vi "Teleop.vi"(10 "Match Info":T1={"Autonomous Elapsed Seconds"=0.0, "TeleOp Elapsed Seconds"=0.0, "Disabled Elapsed Seconds"=0.0, "Visited Autonomous"=FALSE, "Visited TeleOp"=FALSE, "Visited Disabled"=FALSE, "Autonomous Settings"={"Autonomous Style"=enum."Independent", "VI Refnum"=refnum}}, 11 "Call Context":T2) -> ()   [LabVIEW 2019]
doc: "This VI is called for each TeleOp packet received from the DS where the robot is not disabled. It is often used to read from the joysticks and update I/O or to update setpoints for timed control loops. It should complete and return within 20 milliseconds or it may miss DS packets."
uses:
  <vilib>/Rock Robotics/WPI/DriverStation/WPI_DriverStationDerivedRobotMode.ctl
  <vilib>/Rock Robotics/WPI/DriverStation/WPI_DriverStationMatch Info.ctl
  <vilib>/Rock Robotics/WPI/ThirdParty/Phoenix-LabVIEW/Motor Controller/Controls/CTRE_Phoenix_MotorControl_ControlMode.ctl
  <vilib>/Rock Robotics/WPI/Solenoid/WPI_SolenoidValue.ctl
  <vilib>/Rock Robotics/WPI/Utilities/WPI_GetSetVariantRefNum.vi
  <vilib>/Rock Robotics/Network Tables/NT Read Number.vi
  <vilib>/addons/control/pid/pid.llb/PID (DBL).vi
  <vilib>/Rock Robotics/Network Tables/NT Write Number.vi
  <vilib>/Rock Robotics/WPI/ThirdParty/Phoenix-LabVIEW/Motor Controller/Get/CTRE_Phoenix_MotorController_GetSelectedSensorData.vi
  <vilib>/Rock Robotics/Network Tables/NT Write Boolean.vi
  <vilib>/functionblocks/Bistables/SR Bistable/SR Bistable.vi
  <vilib>/Rock Robotics/Network Tables/NT Write Numeric Array.vi
  <vilib>/Rock Robotics/WPI/Solenoid/WPI_SolenoidSetEnum.vi
  <vilib>/functionblocks/FB Core/FB Core.xnode
  <vilib>/Rock Robotics/Network Tables/NT Read Boolean.vi
  <vilib>/addons/control/pid/NI_PID_pid.lvlib
  <vilib>/functionblocks/NI_FunctionBlock Libraries.lvlib
  <vilib>/Rock Robotics/Network Tables/NT Write Boolean Array.vi
panel:
  out "Sample Slider 0":dbl(slide) scale=0.0..5.0
  out "Sample Boolean 1":bool
  out "Sample Boolean 0":bool
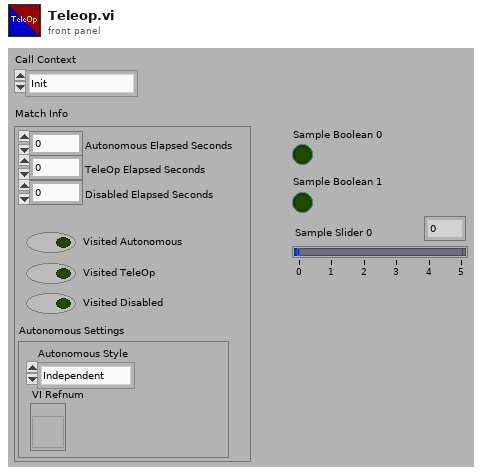
[diagram p1: front panel]
types:
  T1 = typedef "WPI_DriverStationMatch Info.ctl" = cluster{"Autonomous Elapsed Seconds":dbl, "TeleOp Elapsed Seconds":dbl, "Disabled Elapsed Seconds":dbl, "Visited Autonomous":bool, "Visited TeleOp":bool, "Visited Disabled":bool, "Autonomous Settings":cluster{"Autonomous Style":enum16{"Iterative", "Independent"}, "VI Refnum":refnum<vi>}}
  T2 = typedef "WPI_DriverStationDerivedRobotMode.ctl" = enum16{"Init", "Execute", "Stop"}
  T3 = typedef "CTRE_Phoenix_MotorControl_ControlMode.ctl" = u16
  T4 = typedef "WPI_JoystickDevRef.ctl" = cluster{"Device":T5}
  T5 = typedef "WPI_JoystickDeviceEnum.ctl" = enum16{"USB 0", "USB 1", "USB 2", "USB 3", "USB 4", "USB 5"}
  T6 = typedef "WPI_RobotDriveDevRef.ctl" = cluster{"DevStatus":errorcluster, "Motors[]":T7[], "Square Inputs":bool, "Max Output":dbl}
  T7 = typedef "WPI_MotorControlDeviceRef.ctl" = cluster{"DeviceStatus":errorcluster, "Type":T8, "PWM":cluster{"PWM Channel":T9, "DeadBand":T10}, "CAN":cluster{"Device Number":u8, "SetOutput VI Ref":variant, "GetOutput VI Ref":variant, "Enable VI Ref":variant, "Disable VI Ref":variant, "Data":variant}, "Invert":bool, "DIO PWM":cluster{"PWM \"Enable\" Channel":T9, "DIOChannel":T11, "PWM Rate":dbl}}
  T8 = typedef "WPI_MotorControlType.ctl" = enum16{"PWM", "CAN", "DIO PWM"}
  T9 = typedef "FPGA_DIOPWMChannel.ctl" = enum8{"PWM 0", "PWM 1", "PWM 2", "PWM 3", "PWM 4", "PWM 5", "PWM 6", "PWM 7", "PWM 8", "PWM 9", "PWM MXP 0", "PWM MXP 1", "PWM MXP 2", "PWM MXP 3", "PWM MXP 4", "PWM MXP 5", "PWM MXP 6", "PWM MXP 7", "PWM MXP 8", "PWM MXP 9", "Invalid"}
  T10 = typedef "WPI_PWMDeadband.ctl" = cluster{"Name":string, "maxPositivePwm":i32, "minPositivePwm":i32, "centerPwm":i32, "maxNegativePwm":i32, "minNegativePwm":i32, "angularRange":u16}
  T11 = typedef "FPGA_DIOChannel.ctl" = enum8{"DIO 0", "DIO 1", "DIO 2", "DIO 3", "DIO 4", "DIO 5", "DIO 6", "DIO 7", "DIO 8", "DIO 9", "DIO MXP 0", "DIO MXP 1", "DIO MXP 2", "DIO MXP 3", "DIO MXP 4", "DIO MXP 5", "DIO MXP 6", "DIO MXP 7", "DIO MXP 8", "DIO MXP 9", "DIO MXP 10", "DIO MXP 11", "DIO MXP 12", "DIO MXP 13", "DIO MXP 14", "DIO MXP 15", "SPI Port CS1", "SPI Port CS2", "SPI Port CS3", "SPI Port MISO", "SPI Port MOSI", "Invalid"}
  T12 = cluster{"Buttons[0]":bool, "Buttons[1]":bool, "Buttons[2]":bool, "Buttons[3]":bool, "Buttons[4]":bool, "Buttons[5]":bool, "Buttons[6]":bool, "Buttons[7]":bool, "Buttons[8]":bool, "Buttons[9]":bool}
  T13 = cluster{"Axes[0]":dbl, "Axes[1]":dbl, "Axes[2]":dbl, "Axes[3]":dbl, "Axes[4]":dbl, "Axes[5]":dbl, "Axes[6]":dbl, "Axes[7]":dbl, "Axes[8]":dbl}
  T14 = cluster{"proportional gain (Kc)":dbl, "integral time (Ti, min)":dbl, "derivative time (Td, min)":dbl}
  T15 = typedef "WPI_ServoDeviceRef.ctl" = cluster{"DeviceStatus":errorcluster, "PWM Channel":T9, "DeadBand":T10}
  T16 = typedef "WPI_SolenoidDevRef.ctl" = cluster{"DevStatus":errorcluster, "Pneumatics Control Module":u8, "Forward Solenoid Channel":T17, "Reverse Solenoid Channel":T17}
  T17 = typedef "WPI_SolenoidChannel.ctl" = enum8{"Solenoid 0", "Solenoid 1", "Solenoid 2", "Solenoid 3", "Solenoid 4", "Solenoid 5", "Solenoid 6", "Solenoid 7", "Invalid"}
  T18 = typedef "WPI_SolenoidValue.ctl" = enum16{"Off", "On", "Forward", "Reverse"}
  T19 = typedef "WPI_SwitchDevRef.ctl" = cluster{"DevStatus":errorcluster, "DIO Channel":T11, "CntIndex":T20, "Normally Closed":bool}
  T20 = typedef "FPGA_CounterCtrSystemIndex.ctl" = enum8{"Ctr 0", "Ctr 1", "Ctr 2", "Ctr 3", "Ctr 4", "Ctr 5", "Ctr 6", "Ctr 7", "Invalid"}
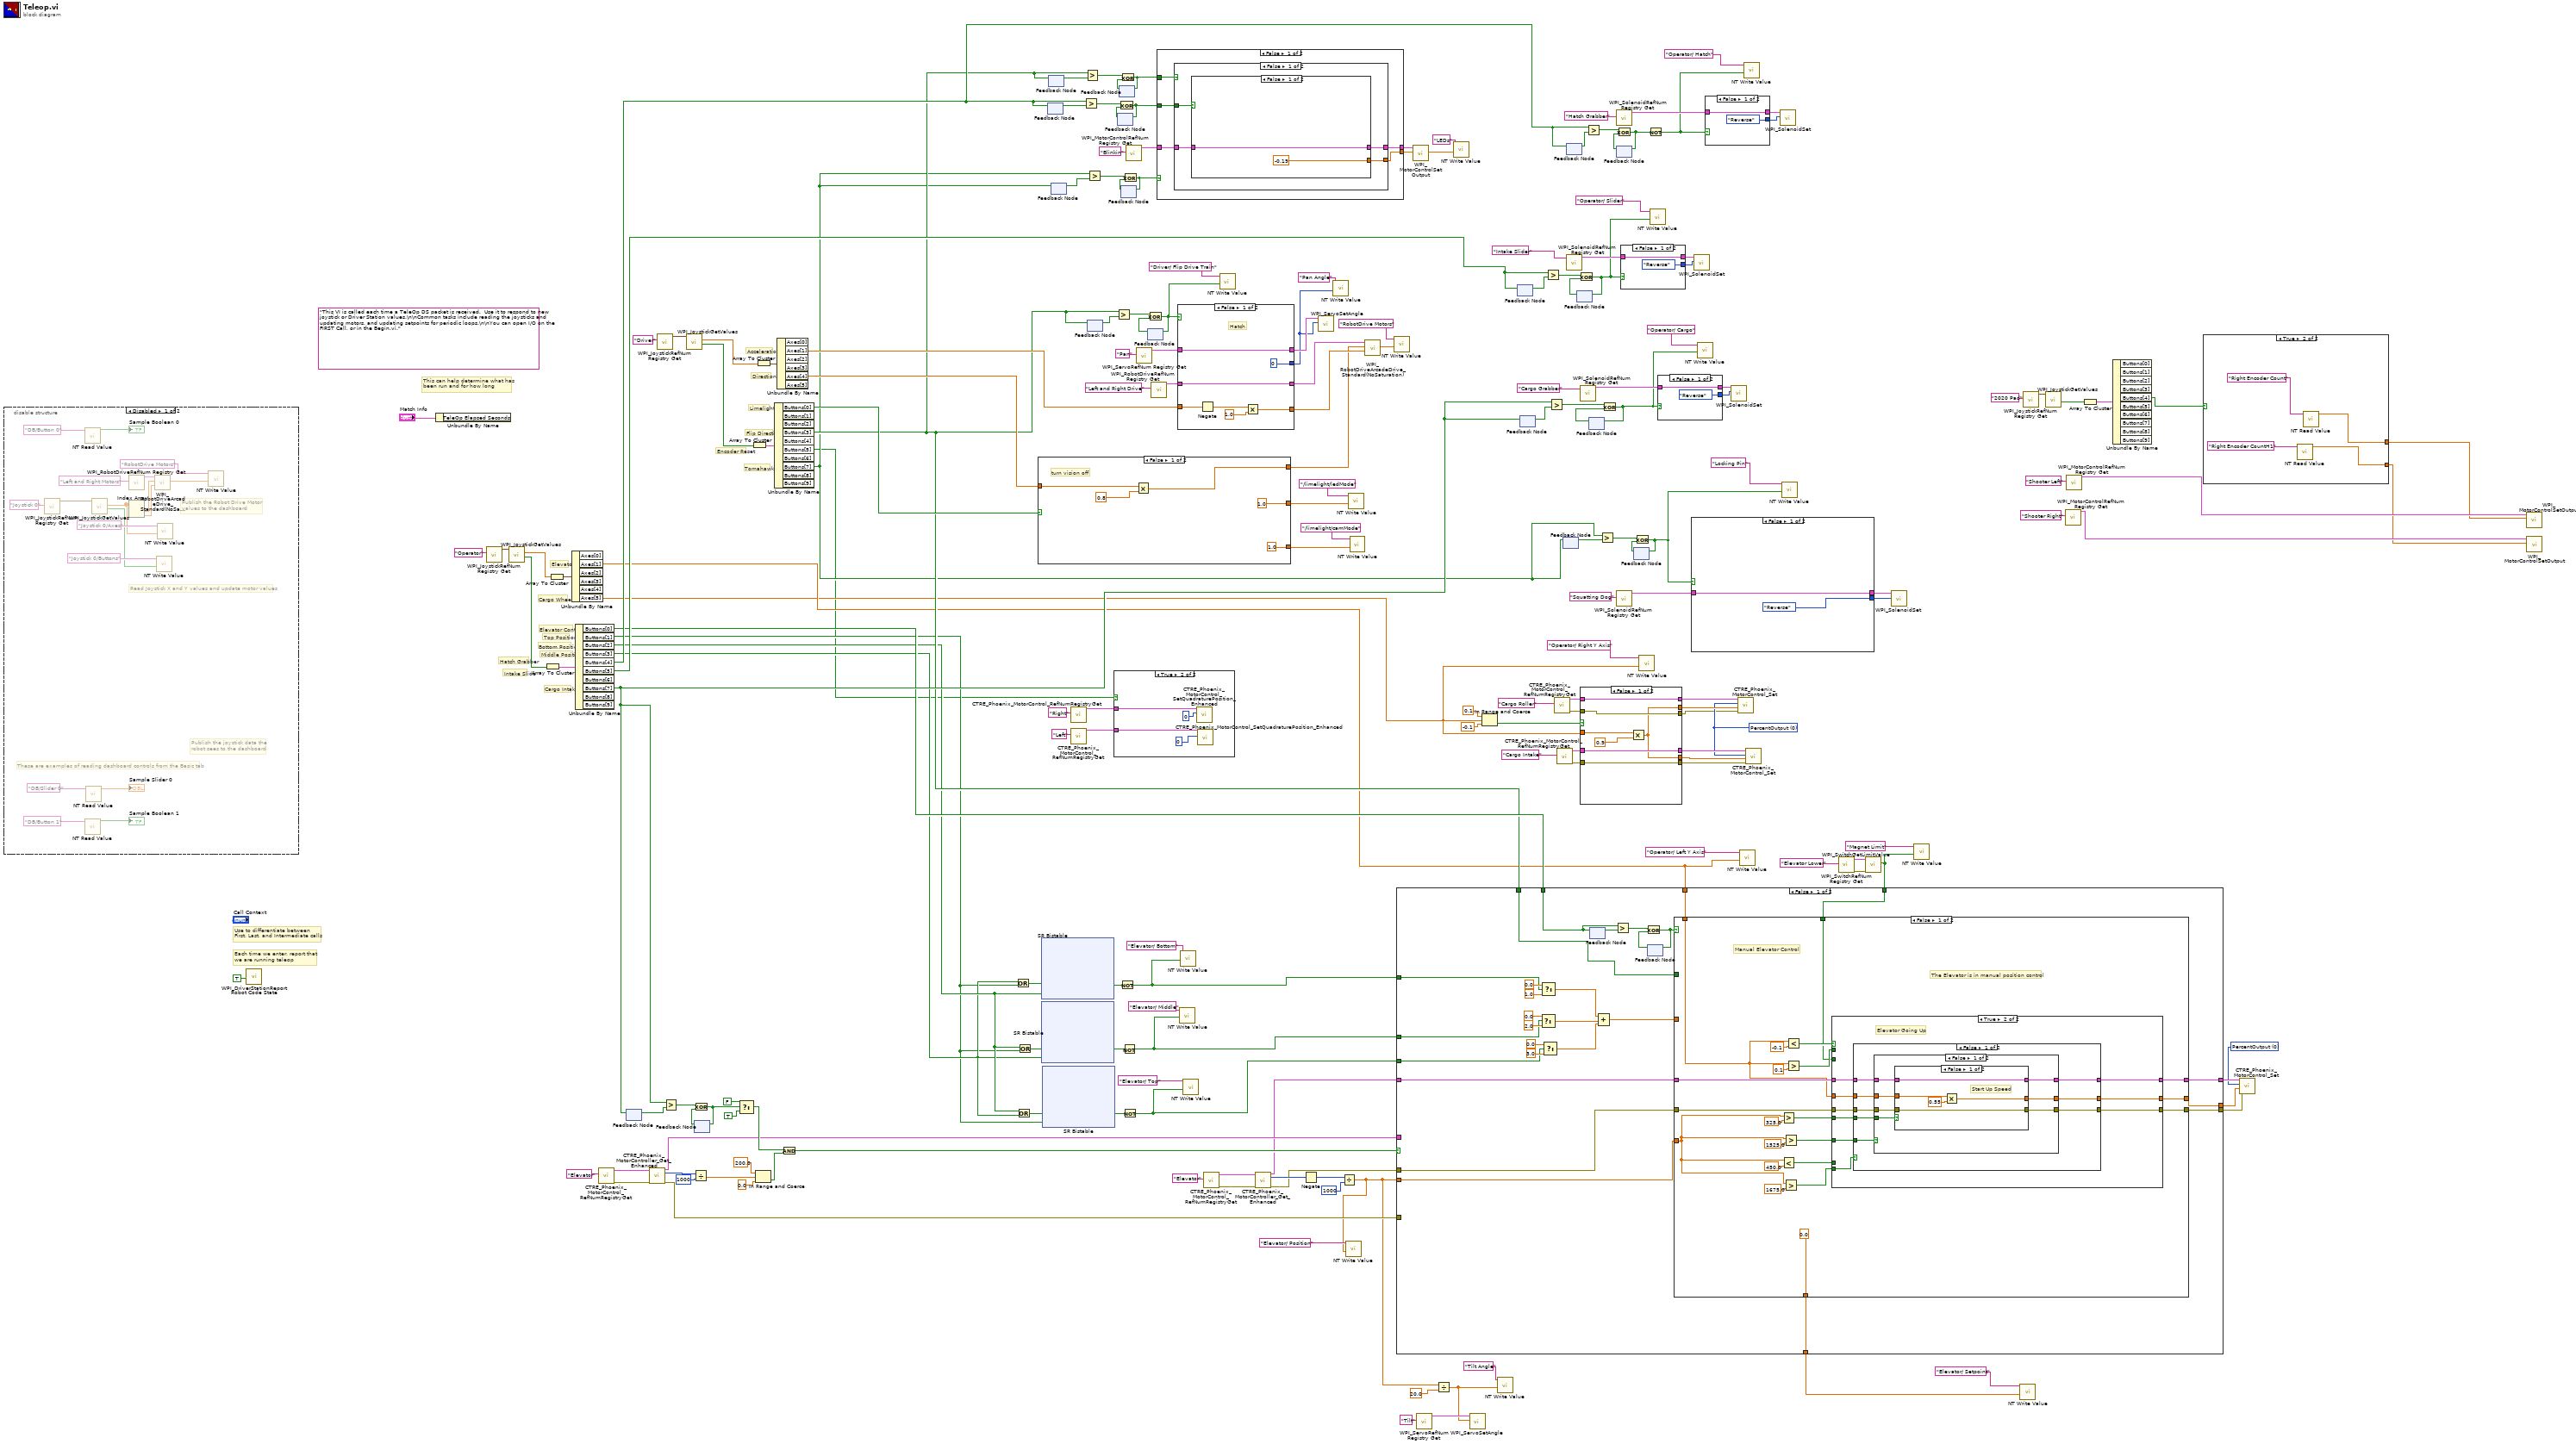
[diagram p0: block diagram]
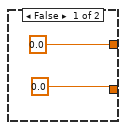
[diagram p2: hidden frame]
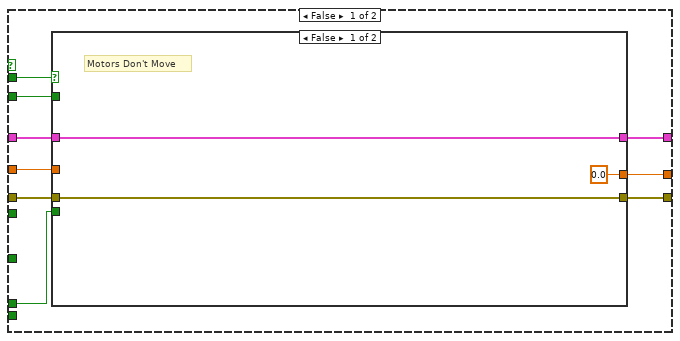
[diagram p4: hidden frame]
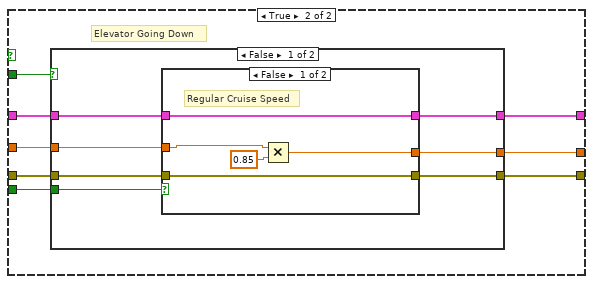
[diagram p5: hidden frame]
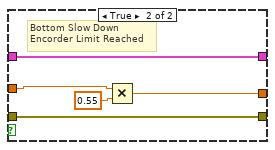
[diagram p6: hidden frame]
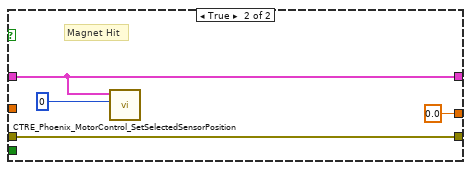
[diagram p7: hidden frame]
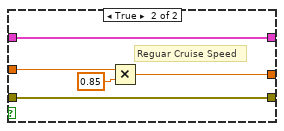
[diagram p8: hidden frame]
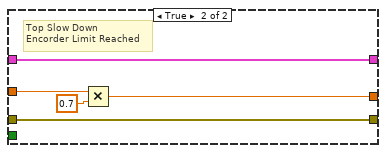
[diagram p9: hidden frame]
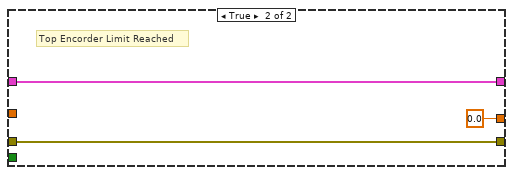
[diagram p10: hidden frame]
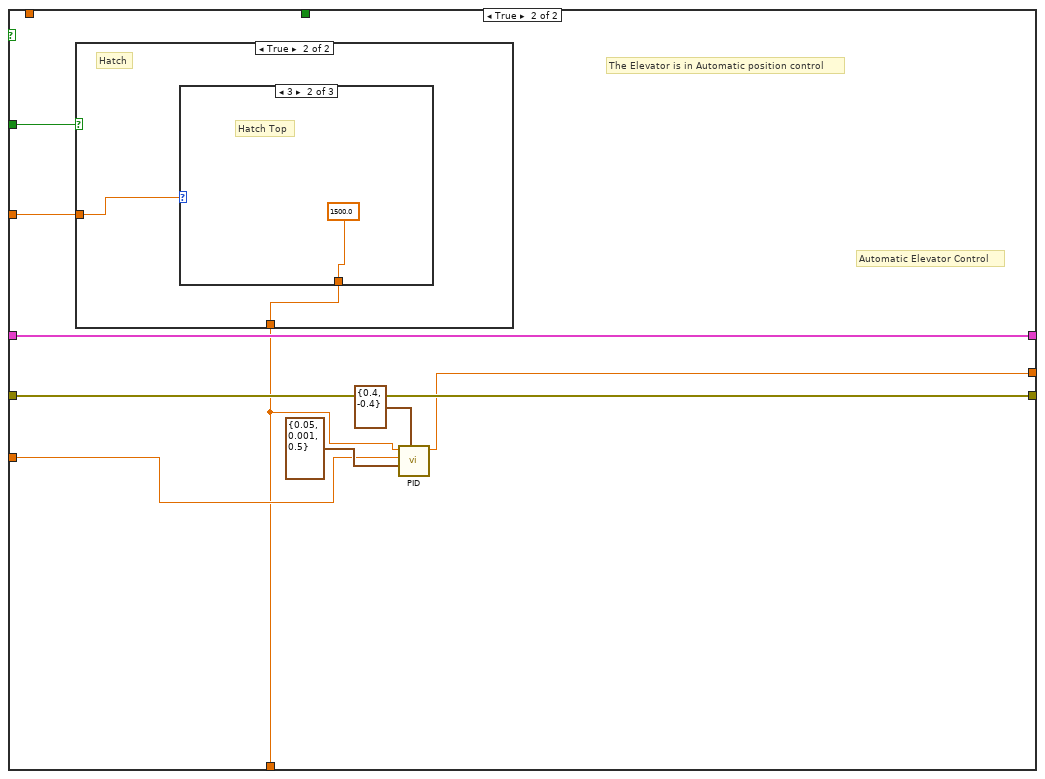
[diagram p11: hidden frame]
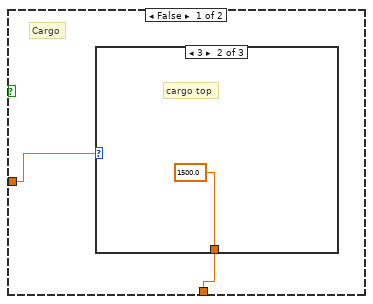
[diagram p12: hidden frame]
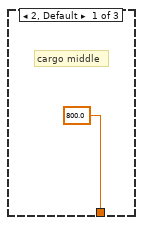
[diagram p13: hidden frame]
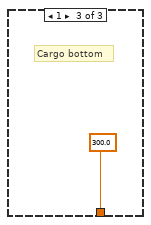
[diagram p14: hidden frame]
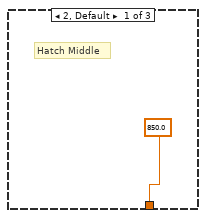
[diagram p15: hidden frame]
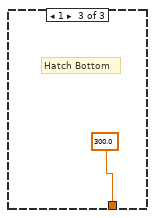
[diagram p16: hidden frame]
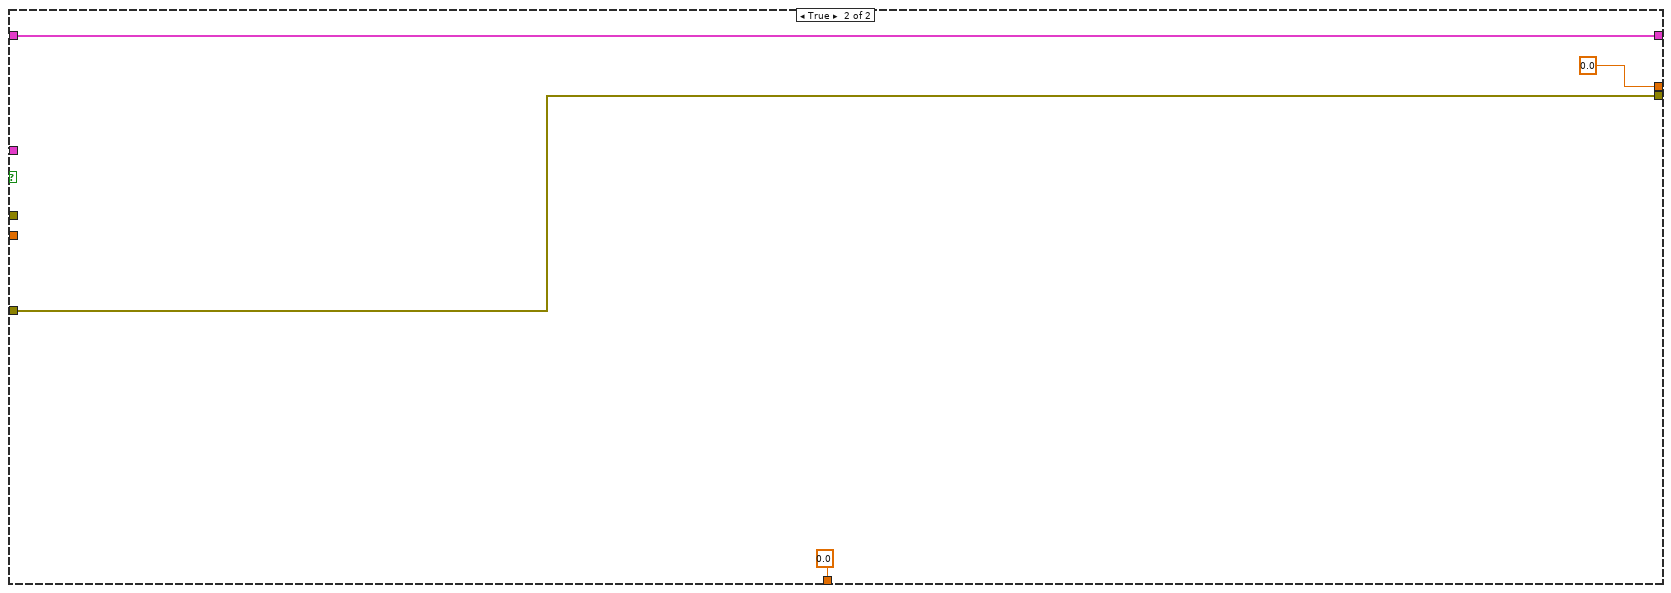
[diagram p17: hidden frame]
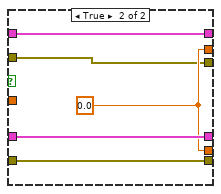
[diagram p18: hidden frame]
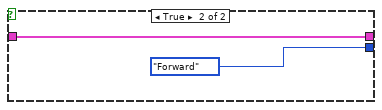
[diagram p19: hidden frame]
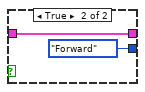
[diagram p20: hidden frame]
diagram:
  w71 = T3 0 items=["PercentOutput"=0, "Position"=1, "Velocity"=2, "Current"=3, "Follower"=5, "MotionProfile"=6, "MotionMagic"=7, "MotionProfileArc"=10, "Disabled"=15] ("Control Mode")
  w95 = T3 0 items=["PercentOutput"=0, "Position"=1, "Velocity"=2, "Current"=3, "Follower"=5, "MotionProfile"=6, "MotionMagic"=7, "MotionProfileArc"=10, "Disabled"=15] ("Control Mode")
  (unwired) "This VI is called each time a TeleOp DS packet is received.  Use it to respond to new joystick or Driver Station values.\n\nCommon tasks include reading the joysticks and updating motors, and updating setpoints for periodic loops.\n\nYou can open I/O on the FIRST Call, or in the Begin.vi."
  # "Acceleration"
  # "Direction"
  # "Limelight"
  # "Flip Direction"
  # "Tomahawks"
  # "Encoder Reset"
  # "Cargo Wheels"
  # "Elevator"
  # "Cargo Intake"
  # "Intake Slide"
  # "Hatch Grabber"
  # "Middle Position"
  # "Bottom Position"
  # "Top Position"
  # "Elevator Control"
  # "Each time we enter, report that\nwe are running teleop"
  # "Use to differentiate between\nFirst, Last, and Intermediate calls"
  # "This can help determine what has\nbeen run and for how long"
  n1 = disable-structure shown="Disabled" {
    frame Disabled {
      # "These are examples of reading dashboard controls from the Basic tab"
      # "Publish the Robot Drive Motor\nvalues to the dashboard"
      # "Publish the joystick data the\nrobot sees to the dashboard"
      # "Read Joystick X and Y values and update motor values"
      n2 = call <vilib>:"WPI_JoystickRefNum Registry Get.vi"("refnum name"="Joystick 0") -> ("JoystickDevRef"=w209:T4)  [unwired: 1 in, 9 out]
      n3 = call-poly <vilib>:"NT Read Value.vi"("Name"="DB/Button 0" ("refnum name")) -> ("Boolean"=→"Sample Boolean 0":bool)  [unwired: 9 in, 1 out]
      n4 = call-poly <vilib>:"NT Read Value.vi"("Name"="DB/Button 1" ("refnum name")) -> ("Boolean"=→"Sample Boolean 1":bool)  [unwired: 9 in, 1 out]
      n5 = call-poly <vilib>:"NT Read Value.vi"("Name"="DB/Slider 0" ("refnum name")) -> ("Numeric"=→"Sample Slider 0":dbl)  [unwired: 9 in, 1 out]
      n6 = call <vilib>:"WPI_JoystickGetValues.vi"("JoystickDevRef"=w209) -> ("Buttons"=w204:bool[], "Axes"=w205:dbl[])  [unwired: 6 in, 3 out]
      n7 = call <vilib>:"WPI_RobotDriveRefNum Registry Get.vi"("refnum name"="Left and Right Motors") -> ("RobotDriveDevRef"=w212:T6)  [unwired: 1 in, 9 out]
      n8 = Index Array(array=w205) -> (element #1=w211:dbl, element #2=w208:dbl)  [unwired: 2 in]
      n9 = call <vilib>:"WPI_RobotDriveArcadeDrive_Standard(NoSaturation).vi"("Y axis value"=w208, "X axis value"=w211, "RobotDriveDevRef"=w212) -> ("Motor Values"=w197:dbl[])  [unwired: 1 in, 7 out]
      n10 = call-poly <vilib>:"NT Write Value.vi"("Boolean Array"=w204, "Name"="Joystick 0/Buttons") -> ()  [unwired: 9 in, 1 out]
      n11 = call-poly <vilib>:"NT Write Value.vi"("Numeric Array"=w205, "Name"="Joystick 0/Axes") -> ()  [unwired: 9 in, 1 out]
      n12 = call-poly <vilib>:"NT Write Value.vi"("Numeric Array"=w197, "Name"="RobotDrive Motors") -> ()  [unwired: 9 in, 1 out]
    }
    frame Enabled {
    }
  }
  n13 = call <vilib>:"WPI_DriverStationReport Robot Code State.vi"("TeleOp"=TRUE ("Autonomous")) -> ()  [unwired: 10 in, 1 out]
  n14 = Unbundle By Name("Match Info") -> ()  [unwired: 1 out]
  n15 = call <vilib>:"WPI_JoystickRefNum Registry Get.vi"("refnum name"="Operator") -> ("JoystickDevRef"=w141:T4)  [unwired: 9 in, 1 out]
  n16 = call <vilib>:"WPI_JoystickGetValues.vi"("JoystickDevRef"=w141) -> ("Buttons"=w144:bool[], "Axes"=w146:dbl[])  [unwired: 6 in, 3 out]
  n17 = Array To Cluster(array=w144) -> (cluster=w143:T12)
  n18 = Array To Cluster(array=w146) -> (cluster=w145:T13)
  n19 = Unbundle By Name(w145) -> ("Axes[1]"=w53:dbl, "Axes[5]"=w14:dbl)  [unwired: 4 out]
  n20 = Unbundle By Name(w143) -> ("Buttons[0]"=w68:bool, "Buttons[1]"=w35:bool, "Buttons[2]"=w37:bool, "Buttons[3]"=w36:bool, "Buttons[4]"=w132:bool, "Buttons[5]"=w122:bool, "Buttons[7]"=w69:bool)  [unwired: 3 out]
  n21 = call <vilib>:"CTRE_Phoenix_MotorControl_RefNumRegistryGet.vi"("refnum name"="Elevator") -> ("error out"=w70:errorcluster, "PhoenixMotorControlDevRef"=w51:T7)  [unwired: 9 in]
  n22 = feedback #1() -> (w87:bool)  [unwired: 1 in]
  n23 = feedback-in #1(w69) -> ()
  n24 = call-poly <vilib>:"CTRE_Phoenix_MotorController_Get_Enhanced.vi"("PhoenixMotorControlDevRef"=w51, "error in"=w70) -> ("PhoenixMotorControlDevRef"=w50:T7, "Position (Raw Sensor Units)"=w77:i32, "error out"=w52:errorcluster)  [unwired: 10 in, 1 out]
  n25 = call <vilib>:"WPI_JoystickRefNum Registry Get.vi"("refnum name"="Driver") -> ("JoystickDevRef"=w168:T4)  [unwired: 9 in, 1 out]
  n26 = Greater?(x=w69, y=w87) -> (0:w88:bool)
  n27 = call <vilib>:"WPI_JoystickGetValues.vi"("JoystickDevRef"=w168) -> ("Buttons"=w191:bool[], "Axes"=w193:dbl[])  [unwired: 6 in, 3 out]
  n28 = Divide(x=w77, y=1000) -> (x/y=w75:dbl)
  n29 = feedback #2() -> (w89:bool)  [unwired: 1 in]
  n30 = Exclusive Or(1:w89, 2:w88) -> (0:w84:bool)
  n31 = feedback-in #2(w84) -> ()
  n32 = Select(t=FALSE, s=w84, f=TRUE) -> (s? t:f=w80:bool)
  n33 = Array To Cluster(array=w191) -> (cluster=w190:T12)
  n34 = Array To Cluster(array=w193) -> (cluster=w192:T13)
  n35 = In Range and Coerce(upper limit=200.0, x=w75, lower limit=0.0) -> (In Range?=w79:bool)  [unwired: 1 out]
  n36 = Unbundle By Name(w190) -> ("Buttons[0]"=w167:bool, "Buttons[3]"=w67:bool, "Buttons[5]"=w12:bool, "Buttons[7]"=w13:bool)  [unwired: 6 out]
  n37 = Unbundle By Name(w192) -> ("Axes[1]"=w165:dbl, "Axes[4]"=w166:dbl)  [unwired: 4 out]
  n38 = And(x=w80, y=w79) -> (x .and. y?=w81:bool)
  n39 = Or(x=w36, y=w35) -> (x .or. y?=w44:bool)
  n40 = Or(x=w37, y=w36) -> (x .or. y?=w46:bool)
  n41 = Or(x=w37, y=w35) -> (x .or. y?=w45:bool)
  n42 = case shown="False" w167 {
    tunnel: [w217 w222] -> w177
    tunnel: [1.0 ("Numeric") 3.0 ("Numeric")] -> w174
    tunnel: [1.0 ("Numeric") 0.0 ("Numeric")] -> w172
    tunnel: w166 -> [w214 _]
    frame False {
      # "turn vision off"
      n43 = Multiply(x=w214, y=0.8) -> (x*y=w217:dbl)
    }
    frame True {
      # "turn vision on"
      n44 = call-poly <vilib>:"NT Read Value.vi"("Name"="/limelight/tx") -> ("Numeric"=w224:dbl)  [unwired: 9 in, 1 out]
      n45 = call-poly <vilib>:"PID.vi"("output range"=cluster{"output high":dbl, "output low":dbl} {"output high"=0.4, "output low"=-0.4}, "PID gains"=T14 {"proportional gain (Kc)"=0.001, "integral time (Ti, min)"=0.001, "derivative time (Td, min)"=0.5}, "process variable"=w224, "setpoint"=0.0) -> ("output"=w222:dbl)  [unwired: 6 in, 1 out]
    }
  }
  n46 = xnode "SR Bistable"("reset"=w44, "set"=w37) -> ("output"=w47:bool)  [unwired: 1 in, 1 out]
  n47 = xnode "SR Bistable"("reset"=w45, "set"=w36) -> ("output"=w48:bool)  [unwired: 1 in, 1 out]
  n48 = xnode "SR Bistable"("reset"=w46, "set"=w35) -> ("output"=w49:bool)  [unwired: 1 in, 1 out]
  n49 = feedback #3() -> (w160:bool)  [unwired: 1 in]
  n50 = feedback-in #3(w132) -> ()
  n51 = feedback #4() -> (w163:bool)  [unwired: 1 in]
  n52 = feedback-in #4(w67) -> ()
  n53 = feedback #5() -> (w150:bool)  [unwired: 1 in]
  n54 = feedback-in #5(w13) -> ()
  n55 = call <vilib>:"CTRE_Phoenix_MotorControl_RefNumRegistryGet.vi"("refnum name"="Right") -> ("PhoenixMotorControlDevRef"=w62:T7)  [unwired: 9 in, 1 out]
  n56 = call <vilib>:"CTRE_Phoenix_MotorControl_RefNumRegistryGet.vi"("refnum name"="Left") -> ("PhoenixMotorControlDevRef"=w60:T7)  [unwired: 9 in, 1 out]
  n57 = Greater?(x=w132, y=w160) -> (0:w159:bool)
  n58 = Greater?(x=w67, y=w163) -> (0:w162:bool)
  n59 = Greater?(x=w13, y=w150) -> (0:w151:bool)
  n60 = feedback #6() -> (w189:bool)  [unwired: 1 in]
  n61 = feedback-in #6(w67) -> ()
  n62 = case shown="True" w12 {
    tunnel: w62 -> [_ w229]
    tunnel: w60 -> [_ w227]
    frame False {
    }
    frame True {
      n63 = call <vilib>:"CTRE_Phoenix_MotorControl_SetQuadraturePosition_Enhanced.vi"("New Position"=0, "PhoenixMotorControlDevRef"=w229) -> ()  [unwired: 8 in, 2 out]
      n64 = call <vilib>:"CTRE_Phoenix_MotorControl_SetQuadraturePosition_Enhanced.vi"("New Position"=0, "PhoenixMotorControlDevRef"=w227) -> ()  [unwired: 8 in, 2 out]
    }
  }
  n65 = Greater?(x=w67, y=w189) -> (0:w188:bool)
  n66 = feedback #7() -> (w158:bool)  [unwired: 1 in]
  n67 = feedback #8() -> (w161:bool)  [unwired: 1 in]
  n68 = Exclusive Or(1:w158, 2:w159) -> (0:w153:bool)
  n69 = feedback-in #7(w153) -> ()
  n70 = Not(x=w47) -> (.not. x?=w40:bool)
  n71 = Exclusive Or(1:w161, 2:w162) -> (0:w157:bool)
  n72 = feedback-in #8(w157) -> ()
  n73 = feedback #9() -> (w152:bool)  [unwired: 1 in]
  n74 = Not(x=w48) -> (.not. x?=w39:bool)
  n75 = Not(x=w49) -> (.not. x?=w38:bool)
  n76 = Exclusive Or(1:w152, 2:w151) -> (0:w149:bool)
  n77 = feedback-in #9(w149) -> ()
  n78 = call <vilib>:"WPI_MotorControlRefNum Registry Get.vi"("refnum name"="Blinkin") -> ("MotorControlDevRef"=w156:T7)  [unwired: 9 in, 1 out]
  n79 = call <vilib>:"WPI_ServoRefNum Registry Get.vi"("refnum name"="Pan") -> ("ServoDeviceRef"=w185:T15)  [unwired: 9 in, 1 out]
  n80 = feedback #10() -> (w187:bool)  [unwired: 1 in]
  n81 = Exclusive Or(1:w187, 2:w188) -> (0:w17:bool)
  n82 = feedback-in #10(w17) -> ()
  n83 = call <vilib>:"WPI_RobotDriveRefNum Registry Get.vi"("refnum name"="Left and Right Drive") -> ("RobotDriveDevRef"=w180:T6)  [unwired: 9 in, 1 out]
  n84 = case shown="False" w149 {
    tunnel: w157 -> [w235 _]
    tunnel: w156 -> [w234 w247]
    tunnel: [w233 w247] -> w155
    tunnel: [w232 -0.57 ("Output")] -> w154
    tunnel: w153 -> [w231 _]
    frame False {
      n85 = case shown="False" w235 {
        tunnel: w234 -> [w238 w245]
        tunnel: [w237 w245] -> w233
        tunnel: [w236 0.63 ("Output")] -> w232
        tunnel: w231 -> [w239 _]
        frame False {
          n86 = case shown="False" w239 {
            tunnel: w238 -> [w241 w243]
            tunnel: [w241 w243] -> w237
            tunnel: [-0.19 ("Output") 0.79 ("Output")] -> w236
            frame False {
            }
            frame True {
            }
          }
        }
        frame True {
        }
      }
    }
    frame True {
    }
  }
  n87 = case shown="False" w17 {
    tunnel: w165 -> [w248 w256]
    tunnel: [w251 w258] -> w178
    tunnel: w185 -> [w254 w260]
    tunnel: [w254 w260] -> w184
    tunnel: [0 ("Angle") 180 ("Angle")] -> w171
    tunnel: w180 -> [w252 w255]
    tunnel: [w252 w255] -> w179
    frame False {
      # "Hatch"
      n88 = Negate(x=w248) -> (-x=w249:dbl)
      n89 = Multiply(x=w249, y=1.0) -> (x*y=w251:dbl)
    }
    frame True {
      # "Cargo"
      n90 = Multiply(x=w256, y=1.0) -> (x*y=w258:dbl)
    }
  }
  n91 = call-poly <vilib>:"NT Write Value.vi"("Boolean"=w39, "Name"="Elevator/ Middle") -> ()  [unwired: 9 in, 1 out]
  n92 = call-poly <vilib>:"NT Write Value.vi"("Boolean"=w40, "Name"="Elevator/ Bottom") -> ()  [unwired: 9 in, 1 out]
  n93 = call-poly <vilib>:"NT Write Value.vi"("Boolean"=w38, "Name"="Elevator/ Top") -> ()  [unwired: 9 in, 1 out]
  n94 = call <vilib>:"CTRE_Phoenix_MotorControl_RefNumRegistryGet.vi"("refnum name"="Elevator") -> ("error out"=w30:errorcluster, "PhoenixMotorControlDevRef"=w27:T7)  [unwired: 9 in]
  n95 = call-poly <vilib>:"NT Write Value.vi"("Boolean"=w17, "Name"="Driver/ Flip Drive Train") -> ()  [unwired: 9 in, 1 out]
  n96 = call-poly <vilib>:"CTRE_Phoenix_MotorController_Get_Enhanced.vi"("PhoenixMotorControlDevRef"=w27, "error in"=w30) -> ("PhoenixMotorControlDevRef"=w29:T7, "Position (Raw Sensor Units)"=w33:i32, "error out"=w28:errorcluster)  [unwired: 10 in, 1 out]
  n97 = Negate(x=w33) -> (-x=w34:i32)
  n98 = call <vilib>:"WPI_ServoSetAngle.vi"("Angle"=w171, "ServoDeviceRef"=w184) -> ()  [unwired: 8 in, 2 out]
  n99 = call-poly <vilib>:"NT Write Value.vi"("Numeric"=w171, "Name"="Pan Angle") -> ()  [unwired: 9 in, 1 out]
  n100 = Divide(x=w34, y=1000) -> (x/y=w20:dbl)
  n101 = call-poly <vilib>:"NT Write Value.vi"("Numeric"=w20, "Name"="Elevator/ Position") -> ()  [unwired: 9 in, 1 out]
  n102 = call-poly <vilib>:"NT Write Value.vi"("Numeric"=w174, "Name"="/limelight/ledMode") -> ()  [unwired: 9 in, 1 out]
  n103 = call-poly <vilib>:"NT Write Value.vi"("Numeric"=w172, "Name"="/limelight/camMode") -> ()  [unwired: 9 in, 1 out]
  n104 = call <vilib>:"WPI_RobotDriveArcadeDrive_Standard(NoSaturation).vi"("Y axis value"=w178, "X axis value"=w177, "RobotDriveDevRef"=w179) -> ("Motor Values"=w183:dbl[])  [unwired: 1 in, 7 out]
  n105 = call-poly <vilib>:"NT Write Value.vi"("Numeric Array"=w183, "Name"="RobotDrive Motors") -> ()  [unwired: 9 in, 1 out]
  n106 = call <vilib>:"WPI_MotorControlSetOutput.vi"("Output"=w154, "MotorControlDevRef"=w155) -> ("Motor Output"=w148:dbl)  [unwired: 7 in, 2 out]
  n107 = call <vilib>:"WPI_ServoRefNum Registry Get.vi"("refnum name"="Tilt") -> ("ServoDeviceRef"=w23:T15)  [unwired: 9 in, 1 out]
  n108 = Divide(x=w20, y=20.0) -> (x/y=w21:dbl)
  n109 = call-poly <vilib>:"NT Write Value.vi"("Numeric"=w148, "Name"="LEDs") -> ()  [unwired: 9 in, 1 out]
  n110 = call <vilib>:"WPI_ServoSetAngle.vi"("Angle"=w21, "ServoDeviceRef"=w23) -> ()  [unwired: 8 in, 2 out]
  n111 = In Range and Coerce(upper limit=0.1, x=w14, lower limit=-0.1) -> (In Range?=w66:bool)  [unwired: 1 out]
  n112 = call-poly <vilib>:"NT Write Value.vi"("Numeric"=w21, "Name"="Tilt Angle") -> ()  [unwired: 9 in, 1 out]
  n113 = feedback #11() -> (w131:bool)  [unwired: 1 in]
  n114 = feedback-in #11(w122) -> ()
  n115 = feedback #12() -> (w115:bool)  [unwired: 1 in]
  n116 = feedback-in #12(w69) -> ()
  n117 = Greater?(x=w122, y=w131) -> (0:w130:bool)
  n118 = Greater?(x=w69, y=w115) -> (0:w116:bool)
  n119 = call <vilib>:"CTRE_Phoenix_MotorControl_RefNumRegistryGet.vi"("refnum name"="Cargo Roller") -> ("error out"=w93:errorcluster, "PhoenixMotorControlDevRef"=w101:T7)  [unwired: 9 in]
  n120 = call <vilib>:"CTRE_Phoenix_MotorControl_RefNumRegistryGet.vi"("refnum name"="Cargo Intake") -> ("error out"=w91:errorcluster, "PhoenixMotorControlDevRef"=w96:T7)  [unwired: 9 in]
  n121 = feedback #13() -> (w110:bool)  [unwired: 1 in]
  n122 = feedback-in #13(w13) -> ()
  n123 = call <vilib>:"WPI_SolenoidRefNum Registry Get.vi"("refnum name"="Intake Slider") -> ("SolenoidDevRef"=w127:T16)  [unwired: 9 in, 1 out]
  n124 = feedback #14() -> (w136:bool)  [unwired: 1 in]
  n125 = feedback-in #14(w132) -> ()
  n126 = feedback #15() -> (w129:bool)  [unwired: 1 in]
  n127 = Exclusive Or(1:w129, 2:w130) -> (0:w123:bool)
  n128 = feedback-in #15(w123) -> ()
  n129 = case shown="False" w66 {
    tunnel: w101 -> [w267 w272]
    tunnel: [w267 w272] -> w102
    tunnel: w14 -> [w266 _]
    tunnel: [w261 w270] -> w103
    tunnel: [w264 w271] -> w97
    tunnel: w96 -> [w264 w271]
    tunnel: [w263 w268] -> w94
    tunnel: w93 -> [w263 w268]
    tunnel: [w262 w269] -> w92
    tunnel: w91 -> [w262 w269]
    tunnel: [w261 w270] -> w90
    frame False {
      n130 = Multiply(x=w266, y=0.9) -> (x*y=w261:dbl)
    }
    frame True {
      w270 = 0.0 ("Climb")
    }
  }
  n131 = call <vilib>:"WPI_SolenoidRefNum Registry Get.vi"("refnum name"="Cargo Grabber") -> ("SolenoidDevRef"=w119:T16)  [unwired: 9 in, 1 out]
  n132 = Greater?(x=w132, y=w136) -> (0:w135:bool)
  n133 = feedback #16() -> (w117:bool)  [unwired: 1 in]
  n134 = Greater?(x=w13, y=w110) -> (0:w111:bool)
  n135 = Exclusive Or(1:w117, 2:w116) -> (0:w113:bool)
  n136 = feedback-in #16(w113) -> ()
  n137 = call <vilib>:"WPI_SolenoidRefNum Registry Get.vi"("refnum name"="Squatting Dog") -> ("SolenoidDevRef"=w106:T16)  [unwired: 9 in, 1 out]
  n138 = call <vilib>:"WPI_SolenoidRefNum Registry Get.vi"("refnum name"="Hatch Grabber") -> ("SolenoidDevRef"=w139:T16)  [unwired: 9 in, 1 out]
  n139 = feedback #17() -> (w134:bool)  [unwired: 1 in]
  n140 = Exclusive Or(1:w134, 2:w135) -> (0:w133:bool)
  n141 = feedback-in #17(w133) -> ()
  n142 = case shown="False" w123 {
    tunnel: w127 -> [w274 w276]
    tunnel: [w274 w276] -> w126
    tunnel: [WPI_SolenoidValue."Reverse" ("Value") WPI_SolenoidValue."Forward" ("Value")] -> w125
    frame False {
    }
    frame True {
    }
  }
  n143 = feedback #18() -> (w112:bool)  [unwired: 1 in]
  n144 = Exclusive Or(1:w112, 2:w111) -> (0:w108:bool)
  n145 = feedback-in #18(w108) -> ()
  n146 = call-poly <vilib>:"NT Write Value.vi"("Numeric"=w14, "Name"="Operator/ Right Y Axis") -> ()  [unwired: 9 in, 1 out]
  n147 = Not(x=w133) -> (.not. x?=w15:bool)
  n148 = call-poly <vilib>:"NT Write Value.vi"("Boolean"=w123, "Name"="Operator/ Slider") -> ()  [unwired: 9 in, 1 out]
  n149 = case shown="False" w113 {
    tunnel: w119 -> [w278 w280]
    tunnel: [w278 w280] -> w120
    tunnel: [WPI_SolenoidValue."Reverse" ("Value") WPI_SolenoidValue."Forward" ("Value")] -> w121
    frame False {
    }
    frame True {
    }
  }
  n150 = case shown="False" w108 {
    tunnel: w106 -> [w282 w284]
    tunnel: [w282 w284] -> w105
    tunnel: [WPI_SolenoidValue."Reverse" ("Value") WPI_SolenoidValue."Forward" ("Value")] -> w104
    frame False {
    }
    frame True {
    }
  }
  n151 = call-poly <vilib>:"WPI_SolenoidSet.vi"("Value"=w125, "SolenoidDevRef"=w126) -> ()  [unwired: 8 in, 2 out]
  n152 = call-poly <vilib>:"NT Write Value.vi"("Boolean"=w113, "Name"="Operator/ Cargo") -> ()  [unwired: 9 in, 1 out]
  n153 = case shown="False" w15 {
    tunnel: w139 -> [w286 w288]
    tunnel: [w286 w288] -> w138
    tunnel: [WPI_SolenoidValue."Reverse" ("Value") WPI_SolenoidValue."Forward" ("Value")] -> w137
    frame False {
    }
    frame True {
    }
  }
  n154 = call-poly <vilib>:"WPI_SolenoidSet.vi"("Value"=w121, "SolenoidDevRef"=w120) -> ()  [unwired: 8 in, 2 out]
  n155 = call <vilib>:"CTRE_Phoenix_MotorControl_Set.vi"("error in (no error)"=w94, "Output"=w103, "Control Mode"=w95, "PhoenixMotorControlDevRef"=w102) -> ()  [unwired: 6 in, 2 out]
  n156 = call-poly <vilib>:"NT Write Value.vi"("Numeric"=w53, "Name"="Operator/ Left Y Axis") -> ()  [unwired: 9 in, 1 out]
  n157 = call-poly <vilib>:"NT Write Value.vi"("Boolean"=w15, "Name"="Operator/ Hatch") -> ()  [unwired: 9 in, 1 out]
  n158 = call <vilib>:"CTRE_Phoenix_MotorControl_Set.vi"("error in (no error)"=w92, "Output"=w90, "Control Mode"=w95, "PhoenixMotorControlDevRef"=w97) -> ()  [unwired: 6 in, 2 out]
  n159 = call-poly <vilib>:"WPI_SolenoidSet.vi"("Value"=w137, "SolenoidDevRef"=w138) -> ()  [unwired: 8 in, 2 out]
  n160 = call-poly <vilib>:"NT Write Value.vi"("Boolean"=w108, "Name"="Locking Pin") -> ()  [unwired: 9 in, 1 out]
  n161 = call <vilib>:"WPI_SwitchRefNum Registry Get.vi"("refnum name"="Elevator Lower") -> ("error out"=w59:errorcluster, "SwitchDevRef"=w58:T19)  [unwired: 9 in]
  n162 = call <vilib>:"WPI_SwitchGetLimitValue.vi"("error in (no error)"=w59, "SwitchDevRef"=w58) -> ("Switch Pressed"=w55:bool)  [unwired: 7 in, 2 out]
  n163 = case shown="False" w81 {
    tunnel: [w302 w442] -> w74
    tunnel: [w301 0.0 ("Climb")] -> w73
    tunnel: [w300 w443] -> w72
    tunnel: w50 -> [_ w443]
    tunnel: w52 -> [_ w442]
    tunnel: w68 -> [w299 _]
    tunnel: w67 -> [w298 _]
    tunnel: w53 -> [w297 _]
    tunnel: w55 -> [w296 _]
    tunnel: w40 -> [w295 _]
    tunnel: w39 -> [w294 _]
    tunnel: w38 -> [w293 _]
    tunnel: w20 -> [w292 _]
    tunnel: w28 -> [w291 _]
    tunnel: w29 -> [w290 _]
    tunnel: [w289 0.0 ("setpoint")] -> w19
    frame False {
      n164 = Select(t=0.0, s=w294, f=2.0) -> (s? t:f=w311:dbl)
      n165 = Select(t=0.0, s=w295, f=1.0) -> (s? t:f=w312:dbl)
      n166 = Select(t=0.0, s=w293, f=3.0) -> (s? t:f=w310:dbl)
      n167 = feedback #19() -> (w314:bool)  [unwired: 1 in]
      n168 = feedback-in #19(w299) -> ()
      n169 = Compound Arithmetic op=ADD(w312, w311, w310) -> (w303:dbl)
      n170 = Greater?(x=w299, y=w314) -> (0:w315:bool)
      n171 = feedback #20() -> (w316:bool)  [unwired: 1 in]
      n172 = Exclusive Or(1:w316, 2:w315) -> (0:w313:bool)
      n173 = feedback-in #20(w313) -> ()
      n174 = case shown="False" w313 {
        tunnel: [w335 w421] -> w301
        tunnel: w290 -> [w334 w428]
        tunnel: [w333 w428] -> w300
        tunnel: w291 -> [w332 w427]
        tunnel: [w326 w427] -> w302
        tunnel: w298 -> [_ w426]
        tunnel: w303 -> [_ w425]
        tunnel: w292 -> [w317 w424]
        tunnel: [0.0 ("setpoint") w422] -> w289
        tunnel: w297 -> [w319 _]
        tunnel: w296 -> [w318 _]
        frame False {
          # "The Elevator is in manual position control"
          # "Manual Elevator Control"
          n175 = Greater?(x=w317, y=325.0) -> (0:w323:bool)
          n176 = Less?(x=w317, y=450.0) -> (x < y?=w321:bool)
          n177 = Greater?(x=w317, y=1525.0) -> (0:w325:bool)
          n178 = Greater?(x=w317, y=1675.0) -> (0:w327:bool)
          n179 = Less?(x=w319, y=-0.1) -> (x < y?=w328:bool)
          n180 = Greater?(x=w319, y=0.1) -> (0:w322:bool)
          n181 = case shown="True" w328 {
            tunnel: [w344 w382] -> w335
            tunnel: w334 -> [w342 w385]
            tunnel: [w343 w386] -> w333
            tunnel: w332 -> [w340 w383]
            tunnel: w327 -> [_ w387]
            tunnel: [w341 w384] -> w326
            tunnel: w325 -> [_ w381]
            tunnel: w319 -> [w338 w380]
            tunnel: w323 -> [_ w379]
            tunnel: w322 -> [w346 _]
            tunnel: w318 -> [w345 _]
            tunnel: w321 -> [w339 _]
            frame False {
              n182 = case shown="False" w346 {
                tunnel: w345 -> [_ w357]
                tunnel: [0.0 ("Climb") w356] -> w344
                tunnel: [w349 w355] -> w343
                tunnel: w342 -> [w349 w354]
                tunnel: [w348 w353] -> w341
                tunnel: w340 -> [w348 w352]
                tunnel: w339 -> [_ w351]
                tunnel: w338 -> [_ w350]
                frame False {
                  # "Motors Don't Move"
                }
                frame True {
                  # "Elevator Going Down"
                  n183 = case shown="False" w357 {
                    tunnel: [w363 0.0 ("Climb")] -> w356
                    tunnel: [w361 w375] -> w355
                    tunnel: w354 -> [w360 w375]
                    tunnel: [w359 w377] -> w353
                    tunnel: w352 -> [w358 w377]
                    tunnel: w351 -> [w364 _]
                    tunnel: w350 -> [w362 _]
                    frame False {
                      n184 = case shown="False" w364 {
                        tunnel: [w369 w374] -> w363
                        tunnel: w362 -> [w368 w373]
                        tunnel: [w367 w371] -> w361
                        tunnel: w360 -> [w367 w371]
                        tunnel: [w366 w370] -> w359
                        tunnel: w358 -> [w366 w370]
                        frame False {
                          # "Regular Cruise Speed"
                          n185 = Multiply(x=w368, y=0.85) -> (x*y=w369:dbl)
                        }
                        frame True {
                          # "Bottom Slow Down\nEncorder Limit Reached"
                          n186 = Multiply(x=w373, y=0.55) -> (x*y=w374:dbl)
                        }
                      }
                    }
                    frame True {
                      # "Magnet Hit"
                      n187 = call <vilib>:"CTRE_Phoenix_MotorControl_SetSelectedSensorPosition.vi"("New Sensor Position"=0, "PhoenixMotorControlDevRef"=w375) -> ()  [unwired: 8 in, 2 out]
                    }
                  }
                }
              }
            }
            frame True {
              # "Elevator Going Up"
              n188 = case shown="False" w387 {
                tunnel: [w394 w420] -> w386
                tunnel: w385 -> [w393 w420]
                tunnel: [w392 w419] -> w384
                tunnel: w383 -> [w391 w419]
                tunnel: [w390 0.0 ("Climb")] -> w382
                tunnel: w381 -> [w395 _]
                tunnel: w380 -> [w389 _]
                tunnel: w379 -> [w388 _]
                frame False {
                  n189 = case shown="False" w395 {
                    tunnel: [w399 w417] -> w394
                    tunnel: w393 -> [w398 w417]
                    tunnel: [w397 w416] -> w392
                    tunnel: w391 -> [w396 w416]
                    tunnel: [w401 w415] -> w390
                    tunnel: w389 -> [w400 w414]
                    tunnel: w388 -> [w402 _]
                    frame False {
                      n190 = case shown="False" w402 {
                        tunnel: [w407 w412] -> w401
                        tunnel: w400 -> [w406 w411]
                        tunnel: [w404 w410] -> w399
                        tunnel: w398 -> [w404 w410]
                        tunnel: [w403 w409] -> w397
                        tunnel: w396 -> [w403 w409]
                        frame False {
                          # "Start Up Speed"
                          n191 = Multiply(x=w406, y=0.55) -> (x*y=w407:dbl)
                        }
                        frame True {
                          # "Reguar Cruise Speed"
                          n192 = Multiply(x=w411, y=0.85) -> (x*y=w412:dbl)
                        }
                      }
                    }
                    frame True {
                      # "Top Slow Down\nEncorder Limit Reached"
                      n193 = Multiply(x=w414, y=0.7) -> (x*y=w415:dbl)
                    }
                  }
                }
                frame True {
                  # "Top Encorder Limit Reached"
                }
              }
            }
          }
        }
        frame True {
          # "The Elevator is in Automatic position control"
          # "Automatic Elevator Control"
          n194 = case shown="True" w426 {
            tunnel: w425 -> [w431 w436]
            tunnel: [w430 w435] -> w422
            frame False {
              # "Cargo"
              n195 = case shown="3" w431 {
                tunnel: [800.0 ("setpoint") 1500.0 ("setpoint") 300.0 ("setpoint")] -> w430
                frame 2, Default {
                  # "cargo middle"
                }
                frame 3 {
                  # "cargo top"
                }
                frame 1 {
                  # "Cargo bottom"
                }
              }
            }
            frame True {
              # "Hatch"
              n196 = case shown="3" w436 {
                tunnel: [850.0 ("setpoint") 1500.0 ("setpoint") 300.0 ("setpoint")] -> w435
                frame 2, Default {
                  # "Hatch Middle"
                }
                frame 3 {
                  # "Hatch Top"
                }
                frame 1 {
                  # "Hatch Bottom"
                }
              }
            }
          }
          n197 = call-poly <vilib>:"PID.vi"("output range"=cluster{"output high":dbl, "output low":dbl} {"output high"=0.4, "output low"=-0.4}, "PID gains"=T14 {"proportional gain (Kc)"=0.05, "integral time (Ti, min)"=0.001, "derivative time (Td, min)"=0.5}, "process variable"=w424, "setpoint"=w422) -> ("output"=w421:dbl)  [unwired: 6 in, 1 out]
        }
      }
    }
    frame True {
    }
  }
  n198 = call-poly <vilib>:"WPI_SolenoidSet.vi"("Value"=w104, "SolenoidDevRef"=w105) -> ()  [unwired: 8 in, 2 out]
  n199 = call-poly <vilib>:"NT Write Value.vi"("Boolean"=w55, "Name"="Magnet Limit") -> ()  [unwired: 9 in, 1 out]
  n200 = call-poly <vilib>:"NT Write Value.vi"("Numeric"=w19, "Name"="Elevator/ Setpoint") -> ()  [unwired: 9 in, 1 out]
  n201 = call <vilib>:"WPI_JoystickRefNum Registry Get.vi"("refnum name"="2020 Pad") -> ("JoystickDevRef"=w8:T4)  [unwired: 9 in, 1 out]
  n202 = call <vilib>:"WPI_JoystickGetValues.vi"("JoystickDevRef"=w8) -> ("Buttons"=w11:bool[])  [unwired: 6 in, 4 out]
  n203 = call <vilib>:"WPI_MotorControlRefNum Registry Get.vi"("refnum name"="Shooter Right") -> ("MotorControlDevRef"=w4:T7)  [unwired: 9 in, 1 out]
  n204 = call <vilib>:"WPI_MotorControlRefNum Registry Get.vi"("refnum name"="Shooter Left") -> ("MotorControlDevRef"=w5:T7)  [unwired: 9 in, 1 out]
  n205 = Array To Cluster(array=w11) -> (cluster=w10:T12)
  n206 = Unbundle By Name(w10) -> ("Buttons[4]"=w2:bool)  [unwired: 9 out]
  n207 = case shown="True" w2 {
    tunnel: [0.0 ("Output") w449] -> w3
    tunnel: [0.0 ("Output") w447] -> w1
    frame False {
    }
    frame True {
      n208 = call-poly <vilib>:"NT Read Value.vi"("Name"="Right Encoder CountH1") -> ("Numeric"=w447:dbl)  [unwired: 9 in, 1 out]
      n209 = call-poly <vilib>:"NT Read Value.vi"("Name"="Right Encoder Count") -> ("Numeric"=w449:dbl)  [unwired: 9 in, 1 out]
    }
  }
  n210 = call <vilib>:"CTRE_Phoenix_MotorControl_Set.vi"("error in (no error)"=w74, "Output"=w73, "Control Mode"=w71, "PhoenixMotorControlDevRef"=w72) -> ()  [unwired: 6 in, 2 out]
  n211 = call <vilib>:"WPI_MotorControlSetOutput.vi"("Output"=w3, "MotorControlDevRef"=w5) -> ()  [unwired: 7 in, 3 out]
  n212 = call <vilib>:"WPI_MotorControlSetOutput.vi"("Output"=w1, "MotorControlDevRef"=w4) -> ()  [unwired: 7 in, 3 out]
